vi "Lossless Medical Image Compression.vi"() -> ()   [LabVIEW 2023]
doc: "This example shows the application of the integer wavelet transform (IWT) in lossless image compression.\n\nThe IWT converts integer signal samples or images into integer wavelet coefficients. You can compress these integer coefficients by entropy-based encoding without further quantization. As a result, you can reconstruct the original signal perfectly from a compressed set of IWT coefficients. \n\nThis example uses the WA Integer Wavelet Transform VI to compute the IWT coefficients of an image and reconstructs the image using the WA Inverse Integer Wavelet Transform VI. By comparing the difference between the original image and reconstructed image, this example shows that the IWT can achieve lossless image compression. In real-world compression applications, you can apply entropy-based encoding techniques such as the Huffman coding to the IWT coefficients of an image.\n\n<b>Instructions:</b>\n1) Run this VI.\n2) Select different images and observe the difference between the original and the reconstructed image."
uses:
  <vilib>/addons/Wavelet Analysis/discrete wavelet transform.llb/WA 2D Integer Wavelet Transform.vi
  <vilib>/addons/Wavelet Analysis/discrete wavelet transform.llb/WA Inverse 2D Integer Wavelet Transform.vi
  <vilib>/addons/_Advanced Signal Processing/NI_AdvSigProcWA.lvlib
panel:
  in  "Data":u16(ring)=123 items=["1D Example Data"=100, "-"=101, "Doppler"=102, "HOP"=103, "TF Sine"=104, "Noisy Doppler"=105, "Sea Temperature"=106, "Sp500"=107, "Power Line"=108, "Engine Knocking"=109, "HeaviSine"=110, "Bumps"=111, "Blocks"=112, "Piece Regular"=113, "HypChirps"=114, "LinChirps"=115, "Chirps"=116, "Piece Polynomial"=117, "ECG"=131, "-"=118, "2D Example Data"=119, "-"=120, "Finger Print (Image)"=121, "Iris Flower (Image)"=122, "Mammogram (Image)"=123, "Lake (Image)"=127, "Two Can 1 (Image)"=132, "Two Can 2 (Image)"=133, "Camera Man (Image)"=134]
  out "Max difference":i32 format="%.3p"
  in  "stop":bool
  out "Histogram of IWT Coefficients":cluster{"Axis":dbl[], "Histogram":i32[]}(graph)
  in  "Wavelet":u16(ring)=25 items=["Haar"=13, "bior2_2"=16, "bior4_4 (FBI)"=25]
  out "Reconstructed Image":i32[][](graph)
  out "IWT Coefficients":i32[][](graph)
  out "Original Image":u8[][](graph)
  in  "Levels":i32=3
  # "Overview: Shows the application of the integer wavelet transform (IWT) in lossless image compression.\nRequirements: LabVIEW Full Development System, Advanced Signal Processing Toolkit\nInstructions: \n1. Run this VI.\n2. Select different images and observe the difference between the original and the reconstructed image.\n3. Click Stop to stop the VI."
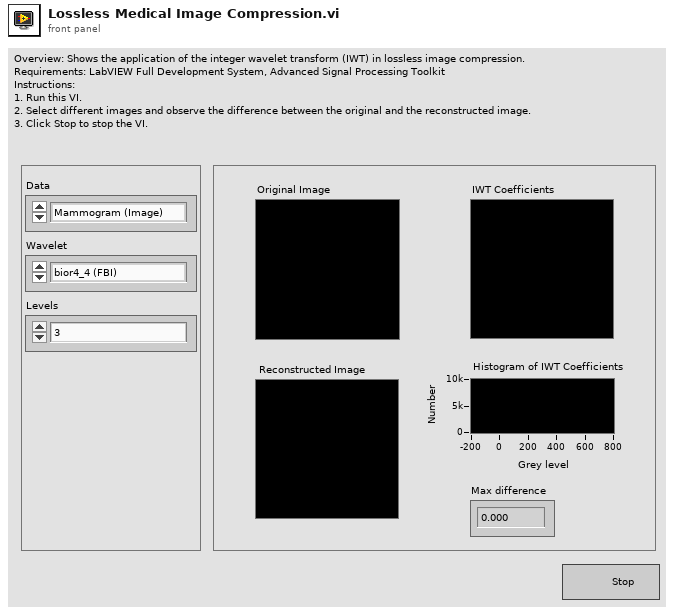
[diagram p1: front panel]
types:
  T1 = cluster{"low_low":i32[][], "low_high":i32[][], "high_low":i32[][], "high_high":i32[][]}[]
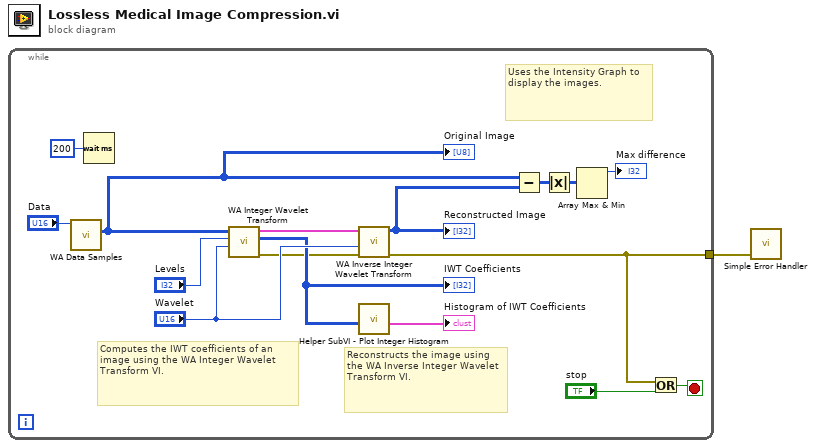
[diagram p0: block diagram]
diagram:
  n1 = while {
    tunnel: [w3] -> w1
    stop <- w11 stop-if-true
    # "Uses the Intensity Graph to display the images."
    # "Reconstructs the image using the WA Inverse Integer Wavelet Transform VI."
    # "Computes the IWT coefficients of an image using the WA Integer Wavelet Transform VI."
    n2 = call <vilib>:"WA Data Samples.vi"("data"="Data") -> ("image"=w9:u8[][])  [unwired: 10 out]
    "Original Image" <- w9
    n3 = Wait (ms)(milliseconds to wait=u32 200 ("millisecond multiple")) -> ()  [unwired: 1 out]
    n4 = call-poly <vilib>:"WA Integer Wavelet Transform.vi"("wavelet"="Wavelet", "levels"="Levels", "signal"=w9) -> ("error out"=w2:errorcluster, "2D IWT plot"=w13:i32[][], "IWT coef"=w16:T1)  [unwired: 1 in, 5 out]
    "IWT Coefficients" <- w13
    n5 = call-poly <vilib>:"WA Inverse Integer Wavelet Transform.vi"("error in (no error)"=w2, "wavelet"="Wavelet", "IWT coef"=w16) -> ("error out"=w3:errorcluster, "signal"=w8:i32[][])  [unwired: 7 out]
    "Reconstructed Image" <- w8
    n6 = call "Helper SubVI - Plot Integer Histogram.vi"("2D integer signal"=w13) -> ("histogram"=→"Histogram of IWT Coefficients":cluster{"x":dbl[], "Histogram":i32[]})  [unwired: 10 in]
    n7 = Subtract(x=w9, y=w8) -> (x-y=w7:i32[][])
    n8 = Absolute Value(x=w7) -> (abs(x)=w6:i32[][])
    n9 = Array Max & Min(array=w6) -> (max value=→"Max difference":i32)  [unwired: 3 out]
    n10 = Or(x=w3, y="stop") -> (x .or. y?=w11:bool)
  }
  n11 = call <vilib>:"Simple Error Handler.vi"("error in (no error)"=w1) -> ()  [unwired: 1 in, 8 out]
